vi "pathplan_vertices_send0.vi"(0 "distance_all":dbl, 1 "angle_all":cdb[](array[numeric]), 3 "数据发送停止开关":bool, 4 "vertices":dbl[][](array[numeric]), 5 "err":dbl[](array[numeric]), 7 "speed_max":dbl[](array[numeric]), 8 "写入串口":refnum<visa-resource-name>, 9 "distance_send_speed":cdb[](array[numeric]), 11 "全场定位串口":refnum<visa-resource-name>="ASRL4::INSTR") -> (20 "路径规划数据写入缓冲区":string, 21 "stop_all":bool)   [LabVIEW 2016]
uses:
  <vilib>/imath/engines/lvmath2/RunTimeEngine/NodeEndStatement/NIMS_NodeEndStatement_Output.vi
  <instcachedir>/0/NIMS_NodeEndStatement_Output_53EC0D466D134D7ABD903AC30B43404B.lvgen/NIMS_NodeEndStatement_Output_53EC0D466D134D7ABD903AC30B43404B_011.vi
  <vilib>/imath/engines/lvmath2/RunTimeEngine/ErrorHandling/NIMS_Finalize Error.vi
  <vilib>/imath/engines/lvmath2/RunTimeEngine/IndexRead/NIMS V(S).vi
  <instcachedir>/0/NIMS V(S)_0488751826AF41519A22953C041130DC.lvgen/NIMS V(S)_0488751826AF41519A22953C041130DC_005.vi
  <vilib>/imath/engines/lvmath2/RunTimeEngine/BuiltInFunctions/abs/NIMS_abs(signed).vi
  <instcachedir>/0/NIMS_abs(signed)_C4FCB8E6058B49B797C7C8D53CA5F6EC.lvgen/NIMS_abs(signed)_C4FCB8E6058B49B797C7C8D53CA5F6EC_008.vi
  <vilib>/imathl/engines/lvmath/Functions/Error Handling/Create Error.vi
  <vilib>/imath/engines/lvmath2/RunTimeEngine/BuiltInFunctions/length/NIMS_length(GM).vi
  <instcachedir>/0/NIMS_length(GM)_47CEC356FCE0482D9BA47DC61C99F2C7.lvgen/NIMS_length(GM)_47CEC356FCE0482D9BA47DC61C99F2C7_000.vi
  <vilib>/imath/engines/lvmath2/RunTimeEngine/RangeToken/NIMS_Range_R2 - Integer.vi
  <instcachedir>/0/NIMS_Range_R2 - Integer_89B873E74E6E489885E44F751DD9C6BF.lvgen/NIMS_Range_R2 - Integer_89B873E74E6E489885E44F751DD9C6BF_000.vi
  <vilib>/imath/engines/lvmath2/RunTimeEngine/CommandStatement/MC_CommandStatement_break.vi
  <instcachedir>/0/NIMS V(S)_0488751826AF41519A22953C041130DC.lvgen/NIMS V(S)_0488751826AF41519A22953C041130DC_000.vi
  <vilib>/imath/engines/lvmath2/RunTimeEngine/IndexRead/NIMS M(S,S).vi
  <instcachedir>/0/NIMS M(S,S)_AC51E74150A542F7991B9634C66F3096.lvgen/NIMS M(S,S)_AC51E74150A542F7991B9634C66F3096_000.vi
  <instcachedir>/0/NIMS_abs(signed)_C4FCB8E6058B49B797C7C8D53CA5F6EC.lvgen/NIMS_abs(signed)_C4FCB8E6058B49B797C7C8D53CA5F6EC_000.vi
  <vilib>/imath/engines/lvmath2/RunTimeEngine/ErrorHandling/NIMS_Create Error From Enums.vi
  <vilib>/imath/engines/lvmath2/RunTimeEngine/IndexRead/NIMS M($,S).vi
  <instcachedir>/0/NIMS M($,S)_3E5749BBB62E49528D4765A77F1F6D98.lvgen/NIMS M($,S)_3E5749BBB62E49528D4765A77F1F6D98_000.vi
  <vilib>/imath/engines/lvmath2/RunTimeEngine/ArithmeticOperatorToken/NIMS_ArithmeticOperator_minus.vi
  <instcachedir>/0/NIMS_ArithmeticOperator_minus_E3B65B1D26A44BB184AFDC5B3F458E3D.lvgen/NIMS_ArithmeticOperator_minus_E3B65B1D26A44BB184AFDC5B3F458E3D_003.vi
  <vilib>/imath/engines/lvmath2/RunTimeEngine/RowToken/NIMS_RowToken_M_CV.vi
  <instcachedir>/0/NIMS_RowToken_M_CV_FA79F1D1D17D44459F3ED8E09EE8B625.lvgen/NIMS_RowToken_M_CV_FA79F1D1D17D44459F3ED8E09EE8B625_000.vi
  <vilib>/imath/engines/lvmath2/RunTimeEngine/RelationalOperatorToken/NIMS_Relational_Operator_Eq.vi
  <instcachedir>/0/NIMS_Relational_Operator_Eq_FD198F059617437A8A02361002FCA645.lvgen/NIMS_Relational_Operator_Eq_FD198F059617437A8A02361002FCA645_006.vi
  <vilib>/imath/engines/lvmath2/RunTimeEngine/BuiltInFunctions/size/NIMS_I32=size(GM,I32).vi
  <instcachedir>/0/NIMS_I32=size(GM,I32)_122058B1B3294FAEA5DC209B92B394E4.lvgen/NIMS_I32=size(GM,I32)_122058B1B3294FAEA5DC209B92B394E4_004.vi
  <vilib>/imath/engines/lvmath2/RunTimeEngine/BuiltInFunctions/norm/NIMS_norm(GV,DBL).vi
  <instcachedir>/0/NIMS_norm(GV,DBL)_1268AFF3C646412B8C6EA3CE75D09042.lvgen/NIMS_norm(GV,DBL)_1268AFF3C646412B8C6EA3CE75D09042_000.vi
  <instcachedir>/0/NIMS_NodeEndStatement_Output_53EC0D466D134D7ABD903AC30B43404B.lvgen/NIMS_NodeEndStatement_Output_53EC0D466D134D7ABD903AC30B43404B_001.vi
  <instcachedir>/0/NIMS_NodeEndStatement_Output_53EC0D466D134D7ABD903AC30B43404B.lvgen/NIMS_NodeEndStatement_Output_53EC0D466D134D7ABD903AC30B43404B_005.vi
  <instcachedir>/0/NIMS_NodeEndStatement_Output_53EC0D466D134D7ABD903AC30B43404B.lvgen/NIMS_NodeEndStatement_Output_53EC0D466D134D7ABD903AC30B43404B_010.vi
  <vilib>/imath/engines/lvmath2/RunTimeEngine/BuiltInFunctions/length/NIMS_length(GV).vi
  <instcachedir>/0/NIMS_length(GV)_08A3D13377FD4E4B96F5795FBF3698FA.lvgen/NIMS_length(GV)_08A3D13377FD4E4B96F5795FBF3698FA_001.vi
  <instcachedir>/0/NIMS V(S)_0488751826AF41519A22953C041130DC.lvgen/NIMS V(S)_0488751826AF41519A22953C041130DC_003.vi
  <vilib>/imath/engines/lvmath2/RunTimeEngine/VariableToken/NIMS_VariableToken_CondDefined.vi
  <instcachedir>/0/NIMS_VariableToken_CondDefined_06E9DA95BD4D46A6BA55EC651A891960.lvgen/NIMS_VariableToken_CondDefined_06E9DA95BD4D46A6BA55EC651A891960_008.vi
  <vilib>/imath/engines/lvmath/Functions/Error Handling/MergeErrorsWrapper.vi
panel:
  out "angle_send":dbl[](array[numeric])
  out "vertices_send":dbl[](array[numeric])
  out "speed_send":dbl[](array[numeric])
  out "错误输出":errorcluster
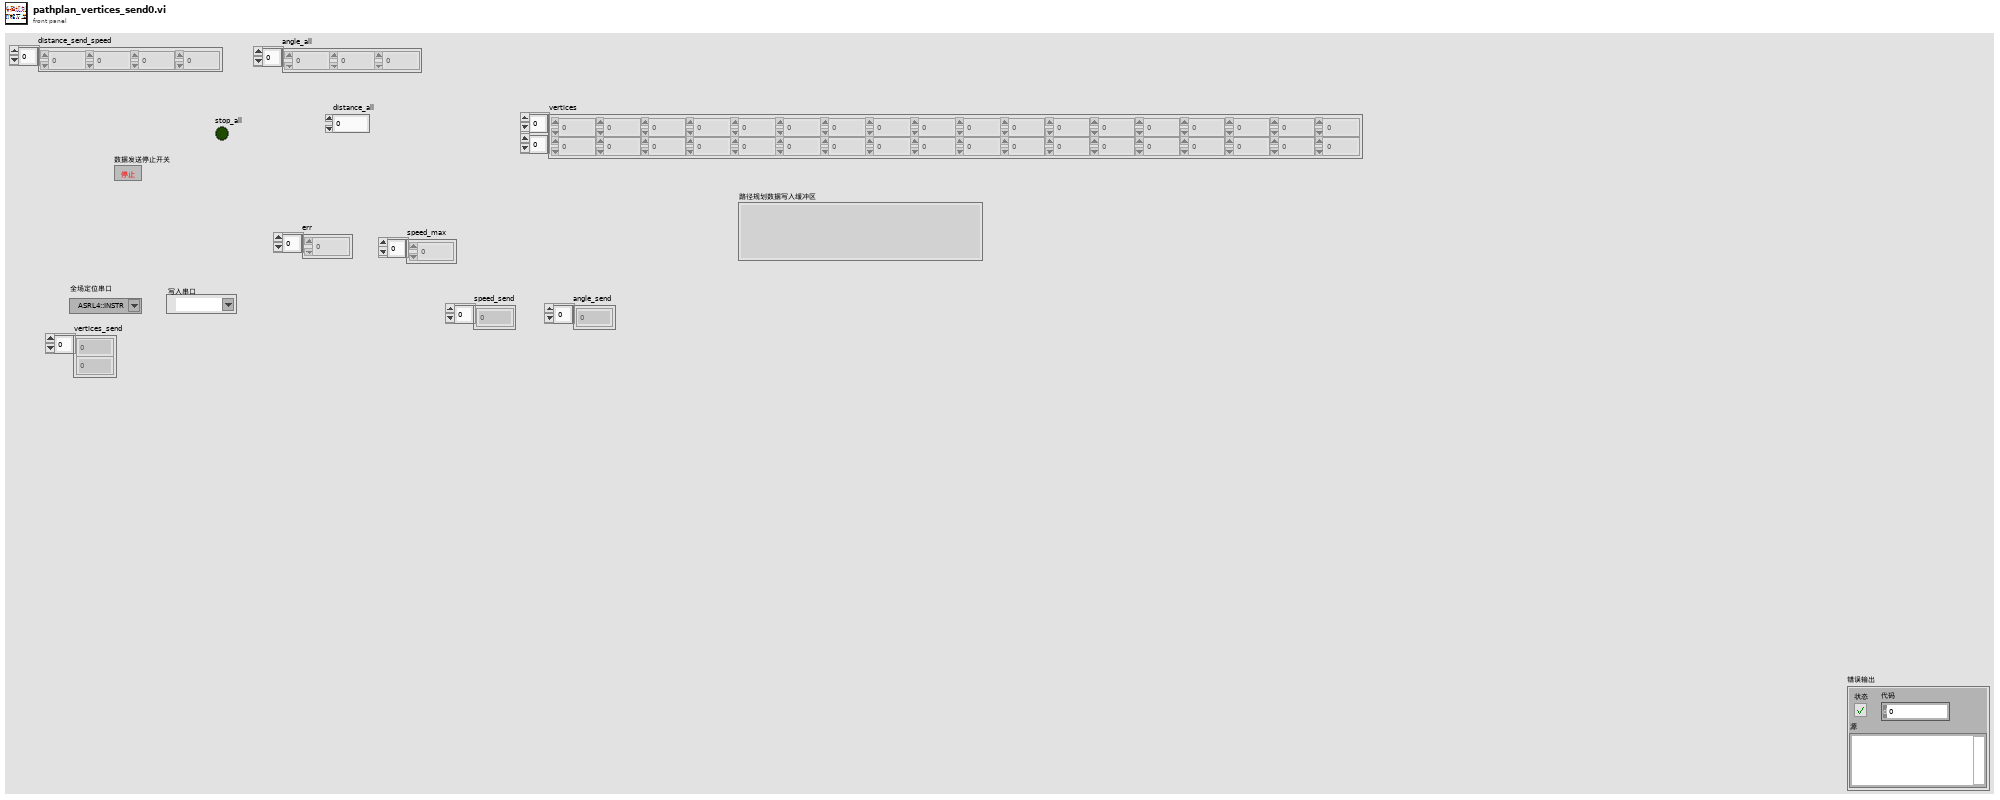
[diagram p1: front panel]
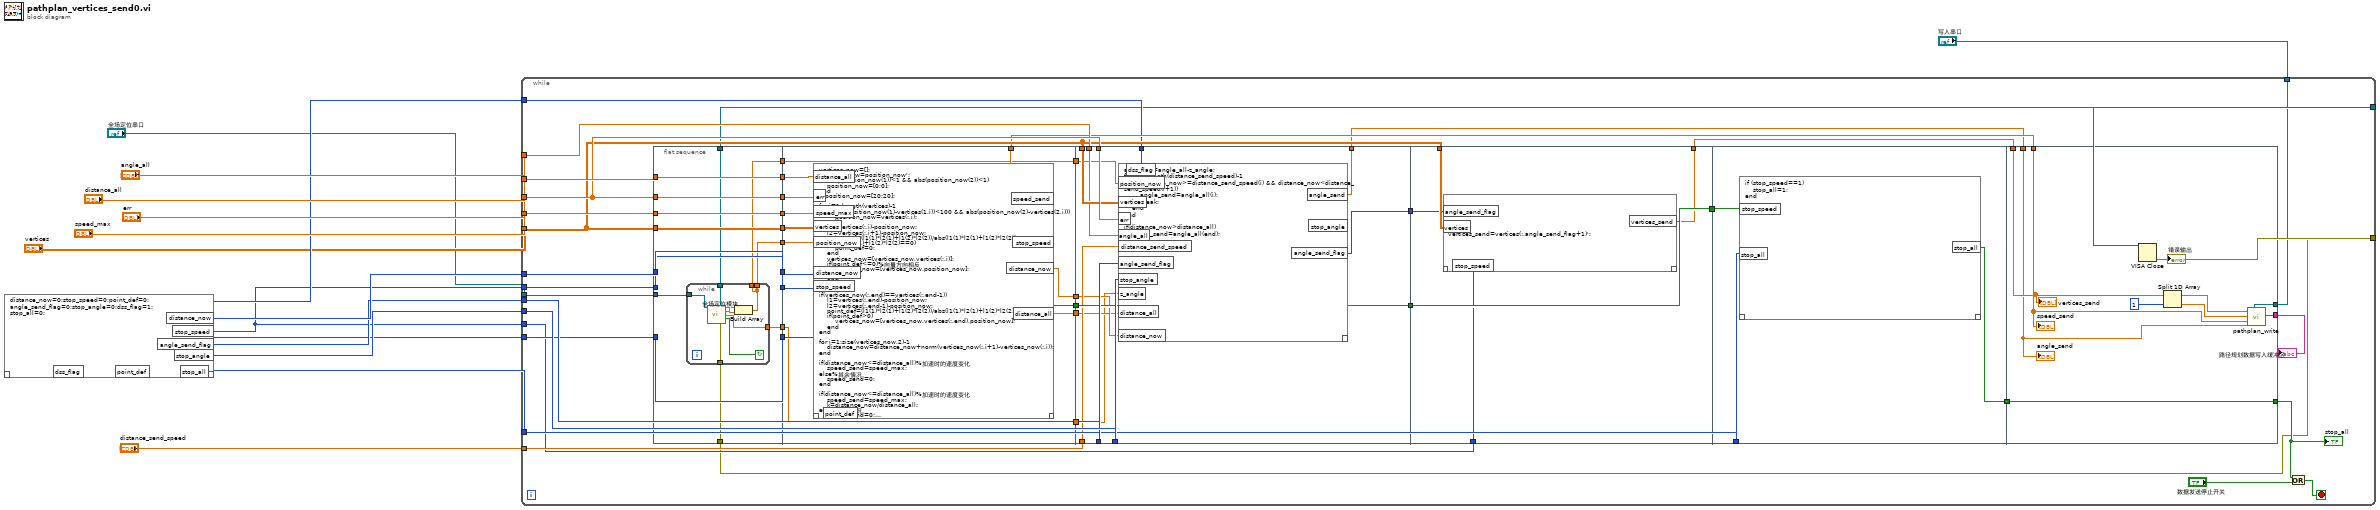
[diagram p0: block diagram]
diagram:
  n1 = mathscript code="distance_now=0;stop_speed=0;point_def=0;\nangle_send_flag=0;stop_angle=0;dss_flag=1;\nstop_all=0;"() -> ("distance_now"=w17:i32, "stop_speed"=w2:i32, "angle_send_flag"=w15:i32, "stop_angle"=w16:i32, "stop_all"=w7:i32, "point_def"=w6:i32, "dss_flag"=w5:i32)  [unwired: 1 in, 1 out]
  n2 = while {
    tunnel: "distance_all" -> [w58]
    tunnel: w17 -> [w57]
    tunnel: w2 -> [w56]
    tunnel: w16 -> [w55]
    tunnel: w15 -> [w54]
    tunnel: "speed_max" -> [w53]
    tunnel: "err" -> [w52]
    tunnel: "angle_all" -> [w51]
    tunnel: "vertices" -> [w50]
    tunnel: [w27] -> w10
    tunnel: [w23] -> w9
    tunnel: "写入串口" -> [w44]
    tunnel: w7 -> [w49]
    tunnel: w6 -> [w39]
    tunnel: "distance_send_speed" -> [w38]
    tunnel: w5 -> [w36]
    tunnel: w2 -> [w35]
    tunnel: "全场定位串口" -> [w22]
    stop <- w42 stop-if-true
    n3 = flat-sequence {
      tunnel: w39 -> [w69]
      tunnel: w50 -> [w70]
      tunnel: w53 -> [w71]
      tunnel: w52 -> [w72]
      tunnel: w56 -> [w73]
      tunnel: w57 -> [w74]
      tunnel: w58 -> [w75]
      tunnel: [w75] -> w34
      tunnel: [w74] -> w33
      tunnel: [w73] -> w32
      tunnel: [w72] -> w31
      tunnel: [w71] -> w30
      tunnel: [w70] -> w29
      tunnel: [w69] -> w28
      tunnel: [w68] -> w27
      tunnel: [w67] -> w26
      tunnel: [w66] -> w24
      tunnel: [w65] -> w23
      tunnel: w22 -> [w64]
      tunnel: [w63] -> w19
      tunnel: [w91] -> w62
      tunnel: [w90] -> w47
      tunnel: [w88] -> w37
      tunnel: w34 -> [w97]
      tunnel: w33 -> [w96]
      tunnel: w32 -> [w95]
      tunnel: w31 -> [w94]
      tunnel: w30 -> [w93]
      tunnel: w29 -> [w92]
      tunnel: w28 -> [w89]
      tunnel: w26 -> [w87]
      tunnel: [w86] -> w25
      tunnel: w24 -> [w86]
      tunnel: [w85] -> w21
      tunnel: [w84] -> w20
      tunnel: w19 -> [w84]
      tunnel: w55 -> [w979]
      tunnel: w54 -> [w978]
      tunnel: w52 -> [w977]
      tunnel: w50 -> [w976]
      tunnel: w51 -> [w975]
      tunnel: [w974] -> w61
      tunnel: [w973] -> w60
      tunnel: w62 -> [w973]
      tunnel: [w972] -> w46
      tunnel: w38 -> [w971]
      tunnel: w37 -> [w970]
      tunnel: w36 -> [w969]
      tunnel: w25 -> [w968]
      tunnel: w21 -> [w967]
      tunnel: w20 -> [w966]
      tunnel: w50 -> [w1215]
      tunnel: w61 -> [w1214]
      tunnel: [w1213] -> w59
      tunnel: w60 -> [w1213]
      tunnel: [w1212] -> w45
      tunnel: w35 -> [w1211]
      tunnel: w59 -> [w1251]
      tunnel: w49 -> [w1252]
      tunnel: [w1253] -> w48
      tunnel: [w1294] -> w43
      tunnel: w48 -> [w1294]
      tunnel: w47 -> [w1290]
      tunnel: w46 -> [w1286]
      tunnel: w45 -> [w1289]
      tunnel: w44 -> [w1288]
      tunnel: [w1287] -> w40
      frame #0 {
        n4 = while {
          tunnel: [w83] -> w68
          tunnel: [w82] -> w67
          tunnel: [w82] -> w66
          tunnel: [w80] -> w65
          tunnel: w64 -> [w79]
          tunnel: [w76] -> w63
          stop <- w81 continue-if-true
          n5 = call "全场定位模块.vi"("VISA resource name"=w79) -> ("VISA资源名称输出"=w83:refnum<visa-resource-name>, "y"=w78:sgl, "x"=w77:sgl, "Zangle"=w76:sgl, "pd"=w81:bool, "错误输出2"=w80:errorcluster)  [unwired: 8 in, 1 out]
          n6 = Build Array(w77, w78) -> (w82:sgl[])
        }
      }
      frame #1 {
        n7 = mathscript code="vertices_now=[];\nposition_now=position_now';\nif (abs(position_now(1))<1 && abs(position_now(2))<1)\n    position_now=[0;0];\nend\n%position_now=[20;20];\n\nfor i=1:length(vertices)-1\n    if(abs(position_now(1)-vertices(1,i))<100 && abs(position_now(2)-vertices(2,i)))\n        position_now=vertices(:,i);\n    end\n    l1=vertices(:,i)-position_now;\n    l2=vertices(:,i+1)-position_now;\n    point_def=(l1(1)*l2(1)+l1(2)*l2(2))/abs(l1(1)*l2(1)+l1(2)*l2(2));\n    if(l1(1)*l2(1)+l1(2)*l2(2)==0)\n        point_def=0;\n    end\n    vertices_now=[vertices_now,vertices(:,i)];\n    if(point_def<=0)%向量方向相反\n        vertices_now=[vertices_now,position_now];\n        break;\n    end\nend\n\nif(vertices_now(:,end)==vertices(:,end-1))\n    l1=vertices(:,end)-position_now;\n    l2=vertices(:,end-1)-position_now;\n    point_def=(l1(1)*l2(1)+l1(2)*l2(2))/abs(l1(1)*l2(1)+l1(2)*l2(2));\n    if(point_def>0)\n        vertices_now=[vertices_now,vertices(:,end),position_now];\n    end\nend\n    \nfor i=1:size(vertices_now,2)-1\n    distance_now=distance_now+norm(vertices_now(:,i+1)-vertices_now(:,i));\nend\n\nif(distance_now<=distance_all)%加速时的速度变化\n    speed_send=speed_max;\nelse%其余情况\n    speed_send=0;\nend\n\nif(distance_now<=distance_all)%加速时的速度变化\n    speed_send=speed_max;\n    k=distance_now/distance_all;\nelse%其余情况\n    speed_send=0;\nend\n\nif(speed_send==0)\n    stop_speed=1;\nend"("err"=w94, "speed_max"=w93, "vertices"=w92, "position_now"=w87, "distance_all"=w97, "distance_now"=w96, "stop_speed"=w95, "point_def"=w89) -> ("stop_speed"=w91:bool, "speed_send"=w90:dbl[], "distance_now"=w88:dbl, "distance_all"=w85:dbl)  [unwired: 1 in, 1 out]
      }
      frame #2 {
        n8 = mathscript code="angle_all=angle_all-z_angle;\nfor i=1:length(distance_send_speed)-1\n    if (distance_now>=distance_send_speed(i) && distance_now<distance_send_speed(i+1))   \n        angle_send=angle_all(i);\n        break;\n    end\nend\n\nif(distance_now>distance_all)\n    angle_send=angle_all(end);\nend"("err"=w977, "angle_all"=w975, "position_now"=w968, "vertices"=w976, "angle_send_flag"=w978, "stop_angle"=w979, "distance_send_speed"=w971, "distance_now"=w970, "dss_flag"=w969, "distance_all"=w967, "z_angle"=w966) -> ("angle_send"=w972:dbl[], "angle_send_flag"=w974:i32)  [unwired: 1 in, 2 out]
      }
      frame #3 {
        n9 = mathscript code="vertices_send=vertices(:,angle_send_flag+1)';"("angle_send_flag"=w1214, "vertices"=w1215, "stop_speed"=w1211) -> ("vertices_send"=w1212:dbl[])  [unwired: 1 in, 1 out]
      }
      frame #4 {
        n10 = mathscript code="if (stop_speed==1)\n    stop_all=1;\nend"("stop_speed"=w1251, "stop_all"=w1252) -> ("stop_all"=w1253:bool)  [unwired: 1 in, 1 out]
      }
      frame #5 {
        n11 = Split 1D Array(array=w1289, index=1 ("索引")) -> (first subarray=w1292:dbl[], second subarray=w1291:dbl[])
        n12 = call "pathplan_write.vi"("VISA资源名称"=w1288, "angle"=w1286, "v"=w1290, "y"=w1291, "x"=w1292) -> ("路径规划数据写入缓冲区"=w1287:string)  [unwired: 6 in]
        "speed_send" <- w1290
        "vertices_send" <- w1289
        "angle_send" <- w1286
      }
    }
    n13 = Or(x=w43, y="数据发送停止开关") -> (x .or. y?=w42:bool)
    "stop_all" <- w43
    "路径规划数据写入缓冲区" <- w40
  }
  n14 = VISA Close(VISA resource name=w10, error in (no error)=w9) -> (error out=→"错误输出":errorcluster)
